vi "Proceed.vi"(7 "component is ready (Y)":bool=TRUE, 8 "error in (no error)":errorcluster, 10 "ProceedMessage":refnum<class "ProceedMessage.lvclass">, 11 "LineCCD in":refnum<class "LineCCD.lvclass">) -> (0 "error out":errorcluster, 2 "all observers are ready?":bool, 3 "LineCCD out":refnum<class "LineCCD.lvclass">)   [LabVIEW 2012, in "LineCCD.lvclass"]
doc: "The Proceed method is used to check if your component is ready. Also it checks if the observers are ready. When the observers and the component are ready, it sends the proceed to its observee. If it's the highest observee, it distributes a stop command."
uses:
  LineCCD.lvclass
  <vilib>/Distrio/Murmex/ProceedMessage/ProceedMessage.lvclass
  LineCCD.lvclass/LineCCD.ctl
  <instrlib>/ALPHALAS CCD S Series/Public/Typedefs/Operating Mode.ctl
  <vilib>/Distrio/Murmex/Murmex/Murmex.lvclass
  <instrlib>/ALPHALAS CCD S Series/ALPHALAS CCD S Series.lvlib
panel:
  # "This method is called when the PROCEED\ntrigger is sent. \n\nOverride this method when your component needs to\nrespond to this trigger. \n\nCall parent for proper implementation"
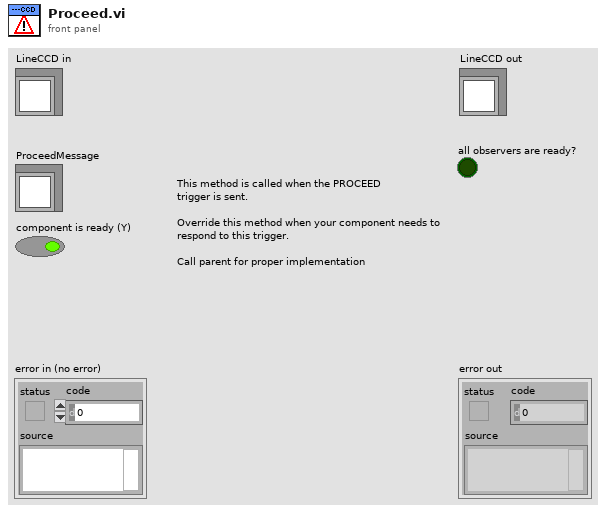
[diagram p1: front panel]
types:
  T1 = typedef "Thorcam.lvclass/imaging mode.ctl" = enum16{"free run mode", "single frame"}
  T2 = typedef "ALPHALAS CCD S Series.lvlib/Operating Mode.ctl" = u16
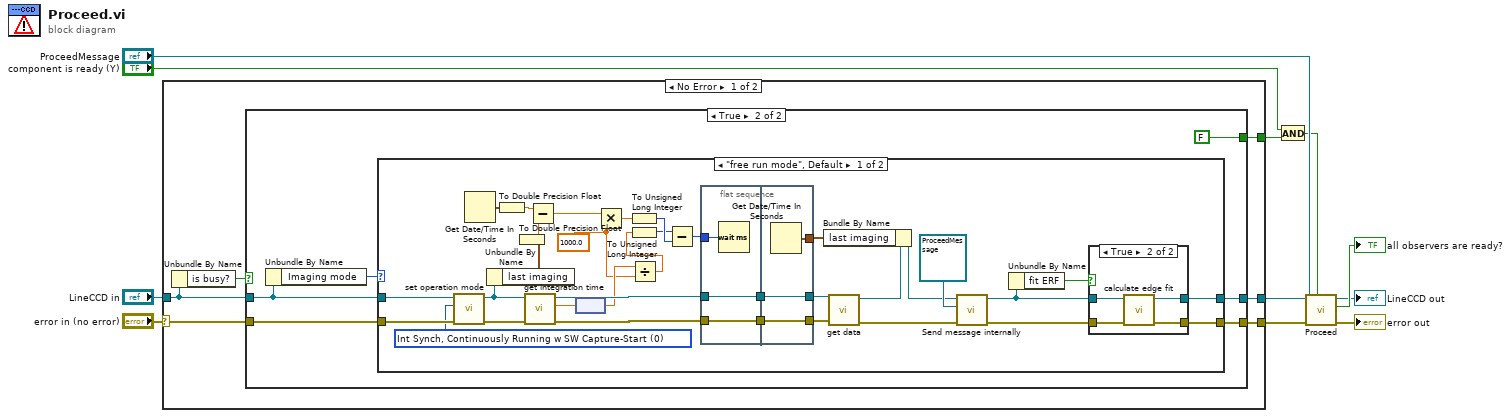
[diagram p0: block diagram]
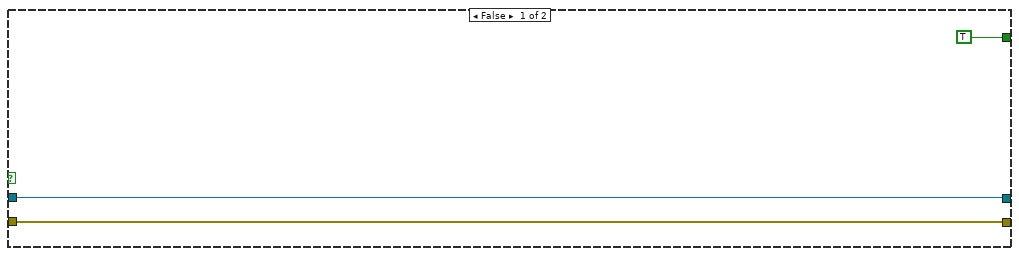
[diagram p2: hidden frame]
diagram:
  n1 = case shown="No Error" "error in (no error)" {
    selector: "error in (no error)" -> [w15 w75]
    tunnel: "LineCCD in" -> [w16 w76]
    tunnel: [w14 w75] -> w6
    tunnel: [w13 w76] -> w5
    tunnel: [w12 _] -> w3
    frame No Error {
      n2 = Unbundle By Name(w16) -> ("is busy?"=w17:bool)
      n3 = case shown="True" w17 {
        tunnel: w16 -> [w19 w26]
        tunnel: w15 -> [w18 w24]
        tunnel: [w18 w23] -> w14
        tunnel: [w19 w22] -> w13
        tunnel: [TRUE FALSE] -> w12
        frame False {
        }
        frame True {
          n4 = Unbundle By Name(w26) -> ("Imaging mode"=w25:T1)
          n5 = case shown="\"free run mode\", Default" w25 {
            tunnel: w26 -> [w37 w74]
            tunnel: w24 -> [w39 w73]
            tunnel: [w30 w74] -> w22
            tunnel: [w29 w73] -> w23
            frame "free run mode", Default {
              w35 = T2 0 items=["Int Synch, Continuously Running w SW Capture-Start", "Int Synch, Continuously Running w HW Capture-Start", "Int Synch, Continuously Running w HW Capture-Enable", "Single Shot, Clean&Ready w ext. HW Trigger", "Ext Synch, Continuously Runnung w SW Capture-Start"] ("Operating Mode (0: Int Synch, Continuously Running w SW Capture-Start)")
              w33 = 1000.0 ("y")
              n6 = call-dynamic "set operation mode.vi"("error in (no error)"=w39, "Operating Mode (0: Int Synch, Continuously Running w SW Capture-Start)"=w35, "LineCCD in"=w37) -> ("error out"=w38:errorcluster, "LineCCD out"=w36:refnum<class "LineCCD.lvclass">)  [unwired: 7 in]
              n7 = Get Date/Time In Seconds() -> (seconds since 1Jan1904=w56:timestamp)
              n8 = Unbundle By Name(w36) -> ("last imaging"=w55:timestamp)
              n9 = To Double Precision Float(number=w56) -> (double precision float=w57:dbl)
              n10 = To Double Precision Float(number=w55) -> (double precision float=w58:dbl)
              n11 = call-dynamic "get integration time.vi"("error in (no error)"=w38, "LineCCD in"=w36) -> ("error out"=w48:errorcluster, "integration time (us)"=w52:dbl[unit], "LineCCD out"=w51:refnum<class "LineCCD.lvclass">)  [unwired: 7 in]
              n12 = Subtract(x=w57, y=w58) -> (x-y=w59:dbl)
              n13 = node(w52) -> (w34:dbl)
              n14 = Multiply(x=w59, y=w33) -> (x*y=w60:dbl)
              n15 = To Unsigned Long Integer(number=w60) -> (unsigned 32bit integer=w54:u32)
              n16 = Divide(x=w34, y=w33) -> (x/y=w32:dbl)
              n17 = To Unsigned Long Integer(number=w32) -> (unsigned 32bit integer=w53:u32)
              n18 = Subtract(x=w53, y=w54) -> (x-y=w45:u32)
              n19 = flat-sequence {
                tunnel: w51 -> [w69]
                tunnel: [w69] -> w50
                tunnel: w48 -> [w68]
                tunnel: [w68] -> w47
                tunnel: w45 -> [w67]
                tunnel: w50 -> [w72]
                tunnel: [w72] -> w49
                tunnel: w47 -> [w71]
                tunnel: [w71] -> w46
                tunnel: [w70] -> w43
                frame #0 {
                  n20 = Wait (ms)(milliseconds to wait=w67) -> ()  [unwired: 1 out]
                }
                frame #1 {
                  n21 = Get Date/Time In Seconds() -> (seconds since 1Jan1904=w70:timestamp)
                }
              }
              n22 = call-dynamic "get data.vi"("error in (no error)"=w46, "LineCCD in"=w49) -> ("error out"=w41:errorcluster, "LineCCD out"=w44:refnum<class "LineCCD.lvclass">)  [unwired: 8 in]
              n23 = Bundle By Name(cluster=w44, "last imaging"=w43) -> (w40:refnum<class "LineCCD.lvclass">)
              n24 = call <vilib>:"Send message internally.vi"("error in (no error)"=w41, "Message"=refnum<class "ProceedMessage.lvclass"> refnum ("Distrio Murmex 1.5:ProceedMessage"), "Murmex in"=w40) -> ("error out"=w31:errorcluster, "Murmex out"=w28:refnum<class "LineCCD.lvclass">)  [unwired: 7 in]
              n25 = Unbundle By Name(w28) -> ("fit ERF"=w27:bool)
              n26 = case shown="True" w27 {
                tunnel: w31 -> [w61 w66]
                tunnel: w28 -> [w62 w65]
                tunnel: [w62 w64] -> w30
                tunnel: [w61 w63] -> w29
                frame False {
                }
                frame True {
                  n27 = call-dynamic "calculate edge fit.vi"("error in (no error)"=w66, "LineCCD in"=w65) -> ("error out"=w63:errorcluster, "LineCCD out"=w64:refnum<class "LineCCD.lvclass">)  [unwired: 8 in]
                }
              }
            }
            frame "single frame" {
            }
          }
        }
      }
    }
    frame Error {
    }
  }
  n28 = And(x="component is ready (Y)", y=w3) -> (x .and. y?=w1:bool)
  n29 = call-parent "Proceed.vi"("component is ready (Y)"=w1, "error in (no error)"=w6, "ProceedMessage"="ProceedMessage", "Murmex in"=w5) -> ("error out"=→"error out":errorcluster, "all observers are ready?"=→"all observers are ready?":bool, "Murmex out"=→"LineCCD out":refnum<class "LineCCD.lvclass">)  [unwired: 5 in]
